vi "AlliGator Display Current Parameter Map (X,Y, I).vi"(7 "Parameter Map Ctrl Refums":T1, 8 "error in (no error)":errorcluster, 11 "AlliGator Internal Variables DVR":refnum<data-value>) -> (0 "error out":errorcluster, 3 "AlliGator Internal Variables DVR":refnum<data-value>)   [LabVIEW 2021, in "AlliGator Action Engine.lvlib"]
doc: "Displays last mouse position and parameter map value at that location."
uses:
  Action Engine/AlliGator Action Engine.lvlib
  AlliGator Parameter Map Control Refnums.ctl
  Internal Variables/AlliGator Internal Variables v2.ctl
  <vilib>/vision/Image Controls.llb/IMAQ Image.ctl
  Internal Variables/AlliGator Gate Image Set.ctl
  Files/AlliGator FLI Dataset Type.ctl
  Files/AlliGator Data Series Type.ctl
  Dual-Channel Datasets/AlliGator Dataset Channel.ctl
  Settings/AlliGator Gate Arithmetic.ctl
  Source Image/AlliGator Displayed Image.ctl
  Image/Named ROI Description.ctl
  Phasor Graph/AlliGator Decay Metadata v3.ctl
  Decay Analysis/Decay Preprocessing/AlliGator Decay Background Subtraction Info.ctl
  Decay Analysis/Decay Preprocessing/AlliGator Baseline Subtraction Method.ctl
  Graphs/XY Graph/XY Graph Plot Shift Parameters.ctl
  Graphs/XY Graph/XY Graph Plot Shift Method.ctl
  Decay Analysis/Decay Preprocessing/AlliGator Decay Extrapolation Parameters.ctl
  Phasor/Calibration Phasor (m, phi).ctl
  Phasor/Phasor Reference Series.ctl
  Phasor/Phasor Calibration Map v2.ctl
  Phasor/Phasor (g, s).ctl
  Phasor Graph/AlliGator Raw Phasor Plot Data v5.ctl
  Phasor/Phasor Standard Deviation Options.ctl
  Phasor Plot/AlliGator Phasor Multi-Harmonic Data.ctl
  Phasor/Phasor Harmonic Data.ctl
  Decay Fit Parameter Map/AlliGator Decay Fit Options & Parameters v3.ctl
  Fits/IRF(X)PSED/Decay Fit Options v3.ctl
  Fits/Decay Convolution/Decay Model.ctl
  Fits/Residual Type.ctl
  Fits/IRF(X)PSED/Fit Weights Type.ctl
  Fits/Non-linear Fitting Method v2.ctl
  Fits/Fit Calculation Method.ctl
  Fits/Non-linear Fitting Algorithm.ctl
  Decay Analysis/Decay Fit/AlliGator Decay Fit Parameter Constraints 2.ctl
  Fits/IRF(X)PSED/Decay Fit Parameters In List.ctl
  Fits/IRF(X)PSED/MLE Baseline Offset Type.ctl
  Decay Analysis/Decay Preprocessing/AlliGator Decay Preprocessing Parameters.ctl
  Fits/IRF(X)PSED/Decay Fit Parameters & Derived Quantities List v2.ctl
  Fits/IRF(X)PSED/Decay Fit Result Constraint.ctl
  Decay Fit Parameter Map/AlliGator Parameter Maps Data.ctl
  <vilib>/vision/NI_Vision_Development_Module.lvlib
  AlliGator Parameter Map.lvlib
  Phasor/Phasor.lvlib
  Image/Image.lvlib
  Decay Analysis/Decay Preprocessing/AlliGator Decay Preprocessing.lvlib
  Graphs/XY Graph/XY Graph Add-Ons.lvlib
  Phasor Graph/AlliGator Phasor Graph.lvlib
  Files/AlliGator Files.lvlib
  Internal Variables/AlliGator Internal Variables.lvlib
  Phasor Plot/AlliGator Phasor Plot.lvlib
  Source Image/AlliGator Source Image.lvlib
  Fits/Fits.lvlib
  Decay Analysis/Decay Fit/AlliGator Decay Fit.lvlib
  Decay Fit Parameter Map/AlliGator Decay Fit Parameter Map.lvlib
  Settings/AlliGator Settings.lvlib
  Dual-Channel Datasets/AlliGator Dual-Channel Datasets.lvlib
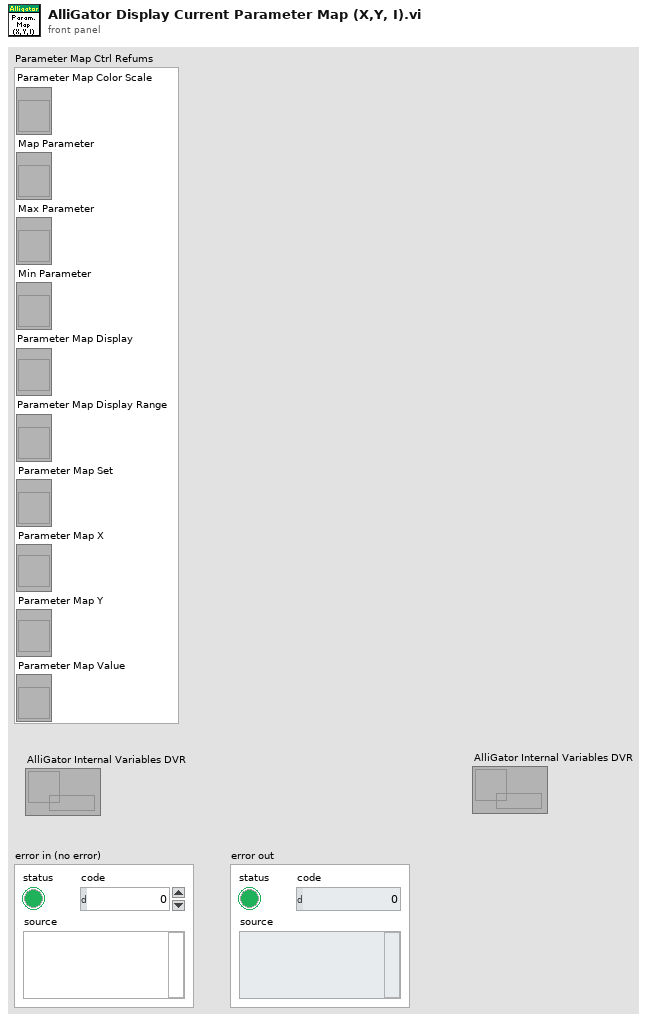
[diagram p1: front panel]
types:
  T1 = typedef "AlliGator Parameter Map.lvlib/AlliGator Parameter Map Control Refnums.ctl" = cluster{"Parameter Map Color Scale":refnum<vi>, "Map Parameter":refnum<vi>, "Max Parameter":refnum<vi>, "Min Parameter":refnum<vi>, "Parameter Map Display":refnum<vi>, "Parameter Map Display Range":refnum<vi>, "Parameter Map Set":refnum<vi>, "Parameter Map X":refnum<vi>, "Parameter Map Y":refnum<vi>, "Parameter Map Value":refnum<vi>}
  T2 = typedef "IMAQ Image.ctl" = refnum<image>
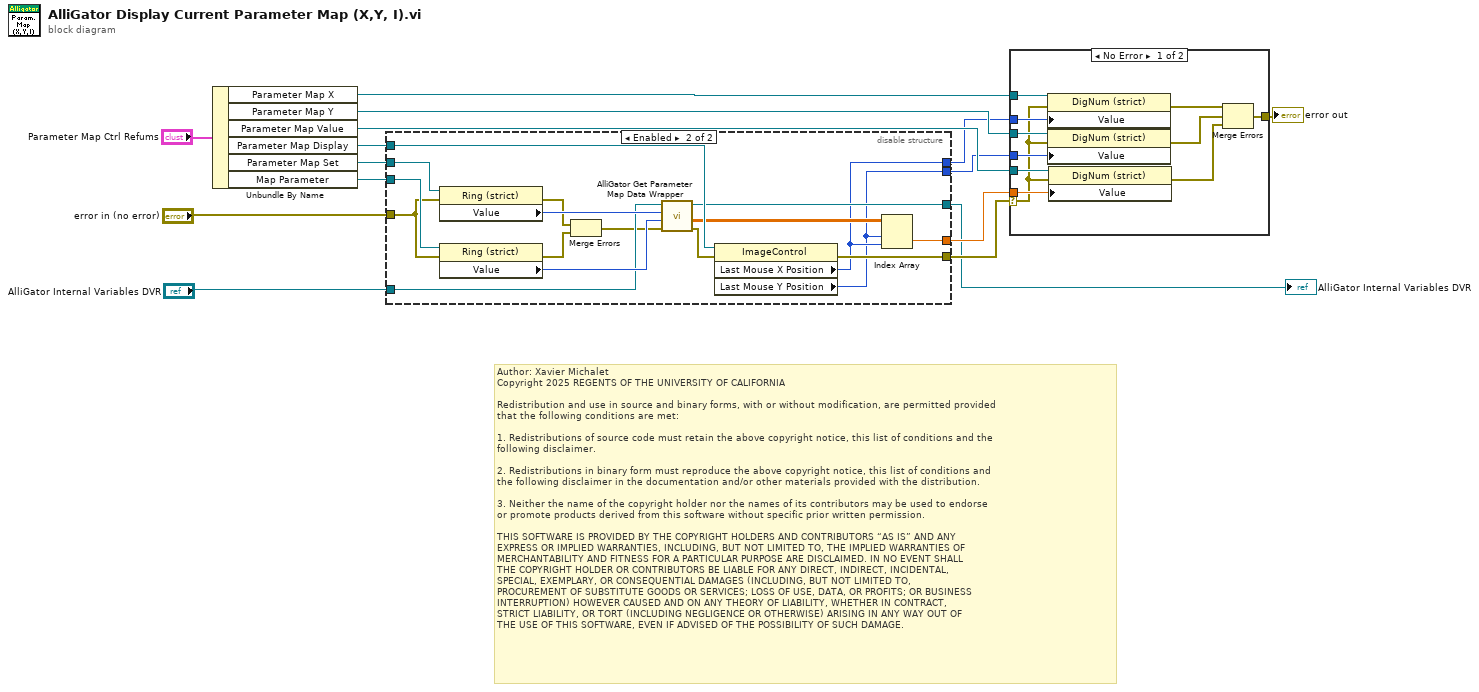
[diagram p0: block diagram]
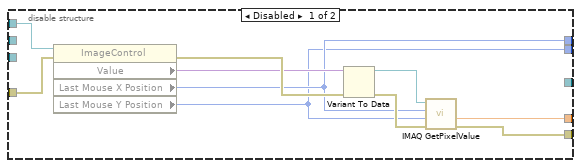
[diagram p2: hidden frame]
diagram:
  # "Author: Xavier Michalet\nCopyright 2025 REGENTS OF THE UNIVERSITY OF CALIFORNIA\n\nRedistribution and use in source and binary forms, with or without modification, are permitted provided\nthat the following conditions are met:\n\n1. Redistributions of source code must retain the above copyright notice, this list of conditions and the\nfollowing disclaimer.\n\n2. Redistributions in binary form must reproduce the above copyright notice, this list of conditions and\nthe following disclaimer in the documentation and/or other materials provided with the distribution.\n\n3. Neither the name of the copyright holder nor the names of its contributors may be used to endorse \nor promote products derived from this software without specific prior written permission.\n\nTHIS SOFTWARE IS PROVIDED BY THE COPYRIGHT HOLDERS AND CONTRIBUTORS “AS IS” AND ANY \nEXPRESS OR IMPLIED WARRANTIES, INCLUDING, BUT NOT LIMITED TO, THE IMPLIED WARRANTIES OF\nMERCHANTABILITY AND FITNESS FOR A PARTICULAR PURPOSE ARE DISCLAIMED. IN NO EVENT SHALL\nTHE COPYRIGHT HOLDER OR CONTRIBUTORS BE LIABLE FOR ANY DIRECT, INDIRECT, INCIDENTAL, \nSPECIAL, EXEMPLARY, OR CONSEQUENTIAL DAMAGES (INCLUDING, BUT NOT LIMITED TO, \nPROCUREMENT OF SUBSTITUTE GOODS OR SERVICES; LOSS OF USE, DATA, OR PROFITS; OR BUSINESS\nINTERRUPTION) HOWEVER CAUSED AND ON ANY THEORY OF LIABILITY, WHETHER IN CONTRACT, \nSTRICT LIABILITY, OR TORT (INCLUDING NEGLIGENCE OR OTHERWISE) ARISING IN ANY WAY OUT OF\nTHE USE OF THIS SOFTWARE, EVEN IF ADVISED OF THE POSSIBILITY OF SUCH DAMAGE."
  n1 = Unbundle By Name("Parameter Map Ctrl Refums") -> ("Parameter Map X"=w14:refnum<vi>, "Parameter Map Y"=w13:refnum<vi>, "Parameter Map Value"=w12:refnum<vi>, "Parameter Map Display"=w10:refnum<vi>, "Parameter Map Set"=w9:refnum<vi>, "Map Parameter"=w8:refnum<vi>)
  n2 = disable-structure shown="Enabled" {
    disable-tunnel: "error in (no error)" -> [w21 w33]
    disable-tunnel: w10 -> [w20 w42]
    disable-tunnel: [w19 w36] -> w4
    disable-tunnel: [w18 w35] -> w3
    disable-tunnel: [w17 w37] -> w5
    disable-tunnel: w8 -> [_ w41]
    disable-tunnel: [_ w40] -> w1
    disable-tunnel: [w16 w38] -> w6
    disable-tunnel: w9 -> [_ w34]
    disable-tunnel: "AlliGator Internal Variables DVR" -> [_ w30]
    frame Disabled {
      n3 = property class="ImageControl"(reference=w20, error in=w21) -> (error out=w24:errorcluster, "Value"=w22:variant, "Last Mouse X Position"=w19:i32, "Last Mouse Y Position"=w18:i32)  [unwired: 1 out]
      n4 = Variant To Data(error in=w24, Variant=w22) -> (data=w23:T2, error out=w25:errorcluster)  [unwired: 1 in]
      n5 = call "IMAQ GetPixelValue"("Image"=w23, "X Coordinate"=w19, "Y Coordinate"=w18, "error in (no error)"=w25) -> ("Pixel Value (Float)"=w16:sgl, "error out"=w17:errorcluster)  [unwired: 2 in, 3 out]
    }
    frame Enabled {
      n6 = property class="Ring (strict)"(reference=w34, error in=w33) -> (error out=w29:errorcluster, "Value"=w32:u16)  [unwired: 1 out]
      n7 = property class="Ring (strict)"(reference=w41, error in=w33) -> (error out=w27:errorcluster, "Value"=w31:u16)  [unwired: 1 out]
      n8 = Merge Errors(w29, w27) -> (w28:errorcluster)
      n9 = call "AlliGator Get Parameter Map Data Wrapper.vi"("error in (no error)"=w28, "Parameter in"=w31, "Map Set"=w32, "Data Value Reference in"=w30) -> ("error out"=w26:errorcluster, "Map Data"=w39:dbl[][], "Data Value Reference out"=w40:refnum<data-value>)  [unwired: 2 in, 3 out]
      n10 = property class="ImageControl"(reference=w42, error in=w26) -> (error out=w37:errorcluster, "Last Mouse X Position"=w36:i32, "Last Mouse Y Position"=w35:i32)  [unwired: 1 out]
      n11 = Index Array(array=w39, index (row)=w35, index (col)=w36) -> (element=w38:dbl)
    }
  }
  "AlliGator Internal Variables DVR" <- w1
  n12 = case shown="No Error" w5 {
    selector: w5 -> [w47 _]
    tunnel: w14 -> [w53 _]
    tunnel: w4 -> [w52 _]
    tunnel: w13 -> [w51 _]
    tunnel: w3 -> [w50 _]
    tunnel: w12 -> [w49 _]
    tunnel: w6 -> [w48 _]
    tunnel: [w43 _] -> w11
    frame No Error {
      n13 = property class="DigNum (strict)"(reference=w53, error in=w47, "Value"=w52) -> (error out=w46:errorcluster)  [unwired: 1 out]
      n14 = property class="DigNum (strict)"(reference=w51, error in=w47, "Value"=w50) -> (error out=w45:errorcluster)  [unwired: 1 out]
      n15 = property class="DigNum (strict)"(reference=w49, error in=w47, "Value"=w48) -> (error out=w44:errorcluster)  [unwired: 1 out]
      n16 = Merge Errors(w46, w45, w44) -> (w43:errorcluster)
    }
    frame Error {
      # "not an image: map is not available"
    }
  }
  "error out" <- w11
